vi "get_tool_from_line.vi"(5 "Drive subsystem name":string, 7 "Tool Assignments":T1, 11 "line in":string) -> (1 "line out":string, 3 "Subsystem out":string)   [LabVIEW 2017, in "labview-standard-library.lvlib" / "automode-scripting.lvlib"]
uses:
  automode-scripting.lvlib
  type-defs/tool-assignments.ctl
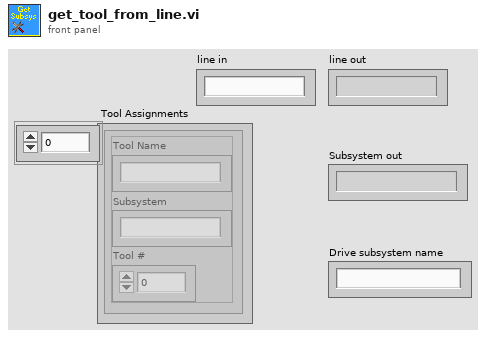
[diagram p1: front panel]
types:
  T1 = typedef "tool-assignments.ctl" = cluster{"Tool Name":string, "Subsystem":string, "Tool #":i32}[]
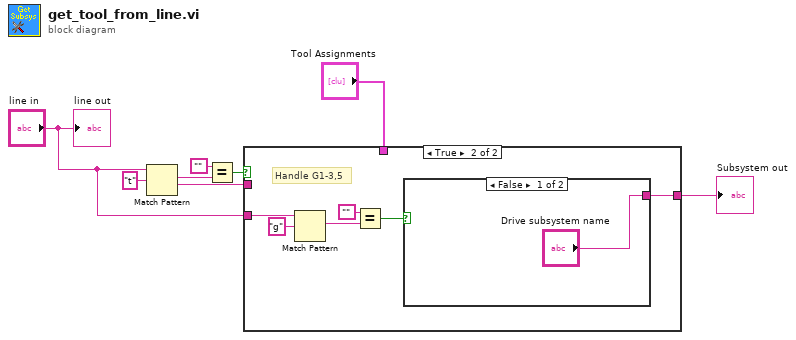
[diagram p0: block diagram]
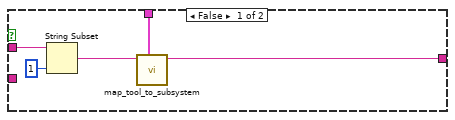
[diagram p2: hidden frame]
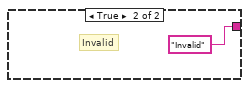
[diagram p3: hidden frame]
diagram:
  n1 = Match Pattern(string="line in", regular expression="t") -> (match substring=w6:string, after substring=w7:string)  [unwired: 1 in, 2 out]
  n2 = Equal?(x="", y=w6) -> (x = y?=w4:bool)
  n3 = case shown="True" w4 {
    tunnel: w7 -> [w13 _]
    tunnel: "Tool Assignments" -> [w11 _]
    tunnel: [w10 w15] -> w2
    tunnel: "line in" -> [_ w17]
    frame False {
      n4 = String Subset(string=w13, length (rest)=1 ("length (rest)")) -> (substring=w9:string)  [unwired: 1 in]
      n5 = call "map_tool_to_subsystem.vi"("Tool Assignments"=w11, "Tool #"=w9) -> ("Subsystem out"=w10:string)  [unwired: 9 in]
    }
    frame True {
      # "Handle G1-3,5"
      n6 = Match Pattern(string=w17, regular expression="g") -> (match substring=w14:string)  [unwired: 1 in, 3 out]
      n7 = Equal?(x="", y=w14) -> (x = y?=w16:bool)
      n8 = case shown="False" w16 {
        tunnel: ["Drive subsystem name" "Invalid"] -> w15
        frame False {
        }
        frame True {
          # "Invalid"
        }
      }
    }
  }
  "Subsystem out" <- w2
  "line out" <- "line in"
